vi "lvlibp_FD_PatternsToExps.vi"(1 "patterns":string="*") -> (0 "array of regular expressions":string[](array[string]))   [LabVIEW 2016]
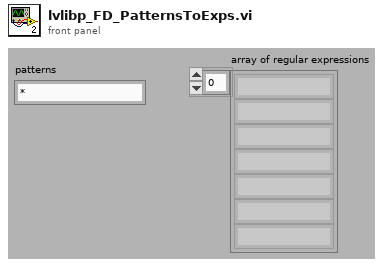
[diagram p1: front panel]
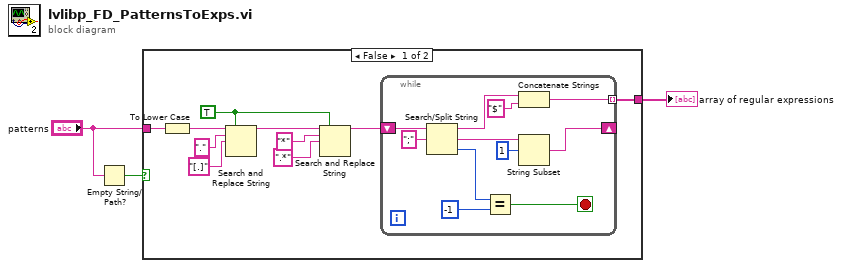
[diagram p0: block diagram]
diagram:
  n1 = Empty String/Path?(string/path="patterns") -> (empty?=w1:bool)
  n2 = case shown="False" w1 {
    tunnel: [w6 _] -> w3
    tunnel: "patterns" -> [w4 _]
    frame False {
      w8 = TRUE ("replace all? (F)")
      n3 = To Lower Case(string=w4) -> (all lower case string=w5:string)
      n4 = Search and Replace String(replace all?=w8, input string=w5, search string=".", replace string="[.]" ("replace string (\"\")")) -> (result string=w11:string)  [unwired: 4 in, 3 out]
      n5 = Search and Replace String(replace all?=w8, input string=w11, search string="*", replace string=".*" ("replace string (\"\")")) -> (result string=w7:string)  [unwired: 4 in, 3 out]
      n6 = while {
        shift-right: [w16] -> _
        shift-left: w7 -> [w23]
        tunnel: [w15] -> w6 mode=indexing
        stop <- w21 stop-if-true
        n7 = Search/Split String(string=w23, search string/char (-)=";") -> (substring before match=w20:string, match + rest of string=w18:string, offset of match=w19:i32)  [unwired: 1 in]
        n8 = Equal?(x=w19, y=-1) -> (x = y?=w21:bool)
        n9 = Concatenate Strings(w20, "$" ("string")) -> (w15:string)
        n10 = String Subset(string=w18, offset (0)=1) -> (substring=w16:string)  [unwired: 1 in]
      }
    }
    frame True {
    }
  }
  "array of regular expressions" <- w3
